vi "Point to Row and Col.vi"(8 "error in (no error)":errorcluster caption="错误输入（无错误）", 10 "点":T2, 11 "Table Ref In":refnum<vi>) -> (0 "error out":errorcluster caption="错误输出", 1 "边界内？":bool, 2 "单元格位置":T1, 3 "Table Ref Out":refnum<vi>)   [LabVIEW 2015]
uses:
  <vilib>/Utility/miscctls.llb/LVPositionTypeDef.ctl
  <vilib>/Utility/miscctls.llb/LVRowAndColumnTypeDef.ctl
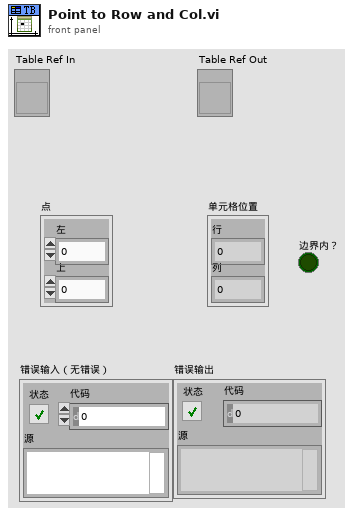
[diagram p1: front panel]
types:
  T1 = typedef "LVRowAndColumnTypeDef.ctl" = cluster{"Row":i32, "Column":i32}
  T2 = typedef "LVPositionTypeDef.ctl" = cluster{"Left":i32, "Top":i32}
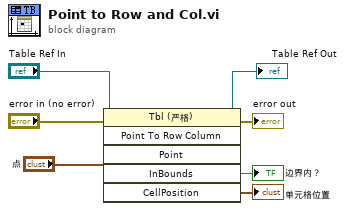
[diagram p0: block diagram]
diagram:
  n1 = invoke class="Tbl (严格)" method="Point To Row Column"(reference="Table Ref In", error in="error in (no error)", "Point"="点") -> (reference out=→"Table Ref Out":refnum<vi>, error out=→"error out":errorcluster, "InBounds"=→"边界内？":bool, "CellPosition"=→"单元格位置":T1)  [unwired: 3 in, 2 out]
